vi "TCP Send Data.vi"(8 "error out":errorcluster, 10 "Clients":refnum<k5>[](array[refnum])) -> (0 "error out":errorcluster, 2 "Clients":refnum<k5>[](array[refnum]), 3 "# of Connections":i32)   [LabVIEW 2020, in "TCP Server.lvlib"]
uses:
  TCP Server.lvlib
panel:
  out "number (0 to 1)":dbl
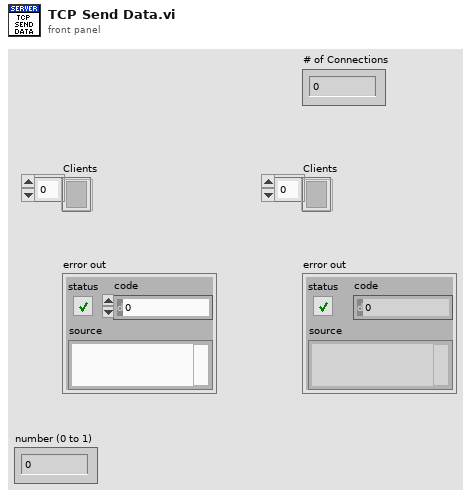
[diagram p1: front panel]
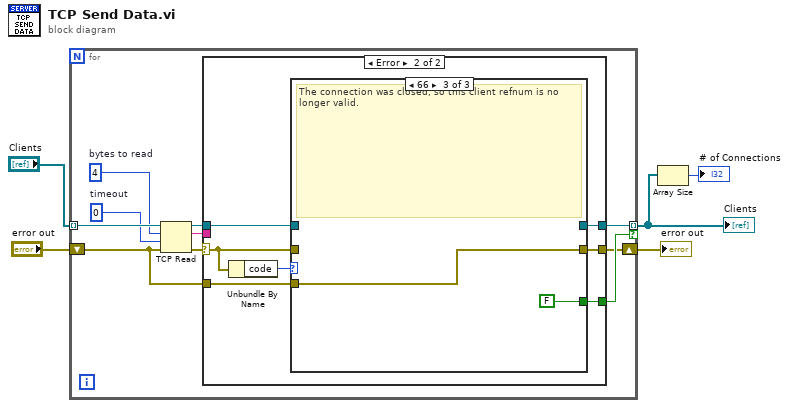
[diagram p0: block diagram]
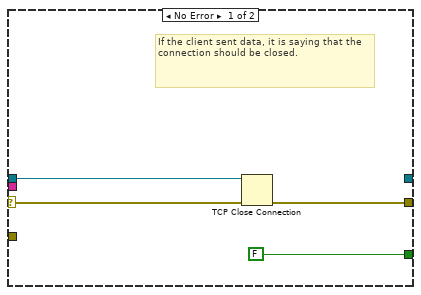
[diagram p2: hidden frame]
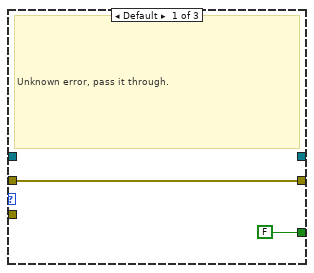
[diagram p3: hidden frame]
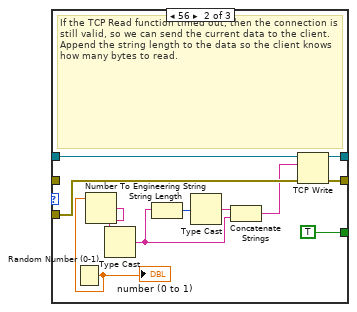
[diagram p4: hidden frame]
diagram:
  n1 = for {
    tunnel: "Clients" -> [w15] mode=indexing
    shift-right: [w7] -> w1
    shift-left: "error out" -> [w6]
    tunnel: [w9] -> w3 mode=indexing if=w8
    w12 = 0  # timeout
    w13 = 4  # bytes to read
    n2 = TCP Read(connection ID=w15, bytes to read=w13, error in (no error)=w6, 9:w12) -> (connection ID out=w14:refnum<k5>, data out=w10:string, error out=w11:errorcluster)  [unwired: 1 out]
    n3 = case shown="Error" w11 {
      selector: w11 -> [w18 w25]
      tunnel: w14 -> [w19 w22]
      tunnel: w10 -> [_ _]
      tunnel: [_ w20] -> w9
      tunnel: [FALSE w21] -> w8
      tunnel: [w16 w24] -> w7
      tunnel: w6 -> [_ w23]
      frame No Error {
        # "If the client sent data, it is saying that the connection should be closed."
        # "If the client sent data, it is saying that the connection should be closed."
        n4 = TCP Close Connection(connection ID=w19, error in (no error)=w18) -> (error out=w16:errorcluster)  [unwired: 2 out]
      }
      frame Error {
        # "Ignore connection closed and timeout errors"
        n5 = Unbundle By Name(w25) -> ("code"=w26:i32)
        n6 = case shown="66" w26 {
          tunnel: w25 -> [w28 _ _]
          tunnel: [w28 w39 w41] -> w24
          tunnel: w23 -> [_ w35 w41]
          tunnel: w22 -> [_ w38 _]
          tunnel: [FALSE TRUE FALSE] -> w21
          tunnel: [_ w37 _] -> w20
          frame Default {
            # "Unknown error, pass it through."
          }
          frame 56 {
            # "If the TCP Read function timed out, then the connection is still valid, so we can send the current data to the client. Append the string length to the data so the client knows how many bytes to read."
            n7 = Random Number (0-1)() -> (number: 0 to 1=w30:dbl)
            "number (0 to 1)" <- w30
            n8 = Number To Engineering String(4:w30) -> (0:w29:string)  [unwired: 3 in]
            n9 = Type Cast(x=w29) -> (*(type *) &x=w31:string)  [unwired: 1 in]
            n10 = String Length(string=w31) -> (length=w33:i32)
            n11 = Type Cast(x=w33) -> (*(type *) &x=w34:string)  [unwired: 1 in]
            n12 = Concatenate Strings(w34, w31) -> (w32:string)
            n13 = TCP Write(connection ID=w38, data in=w32, error in (no error)=w35) -> (connection ID out=w37:refnum<k5>, error out=w39:errorcluster)  [unwired: 2 out]
          }
          frame 66 {
            # "The connection was closed, so this client refnum is no longer valid."
          }
        }
      }
    }
  }
  "Clients" <- w3
  "error out" <- w1
  n14 = Array Size(array=w3) -> (size(s)=→"# of Connections":i32)
